vi "Keyboard MicroDrive Control.vi"() -> ()   [LabVIEW 2020]
uses:
  <vilib>/Utility/inputDevices.llb/keyboardAcquire.vi
  <vilib>/Utility/inputDevices.llb/closeKeyboard.vi
  MicroDrive.dll
panel:
  in  "Move size (um)":dbl=10.0
  in  "M3 Decreasing":string(combo)="16"
  in  "M3 Increasing":string(combo)="29"
  in  "Reset M3":bool
  out "M3-Encoder (um)":dbl format="%.3f"
  out "M3 Reverse Limit":bool
  out "M3 Forward Limit":bool
  in  "stop 2":bool
  in  "Stop":bool
  in  "Move":bool
  in  "Velocity (mm/s)":dbl=1.5 format="%.3f"
  in  "Keyboard Option":bool
  in  "M2 Increasing":string(combo)="32"
  in  "M2 Decreasing":string(combo)="28"
  in  "M1 Decreasing":string(combo)="10"
  in  "M1 Increasing":string(combo)="13"
  out "M1 Reverse Limit":bool
  out "M1 Forward Limit":bool
  out "M2 Reverse Limit":bool
  out "M2 Forward Limit":bool
  in  "Reset M2":bool
  out "M2-Encoder (um)":dbl format="%.3f"
  in  "Reset  All":bool
  in  "Reset M1":bool
  out "M1-Encoder (um)":dbl format="%.3f"
  in  "Move size (Um)":dbl=50.0 format="%.3f"
  in  "Axis":enum16{"M1", "M2", "M3"}(ring)
  in  "MoveMap":string(combo)="11"
  in  "HaltMap":string(combo)="12"
  out "First Key":T1(ring)
  out "keys pressed":T2(array[ring])
  out "Dir Ind":u32(knob) scale=0.0..36.0
  # "Encoder Monitor"
  # "Modified\nfor DM project"
  # "Options"
  # "Keyboard Configuration"
  # "Move without Keyboard"
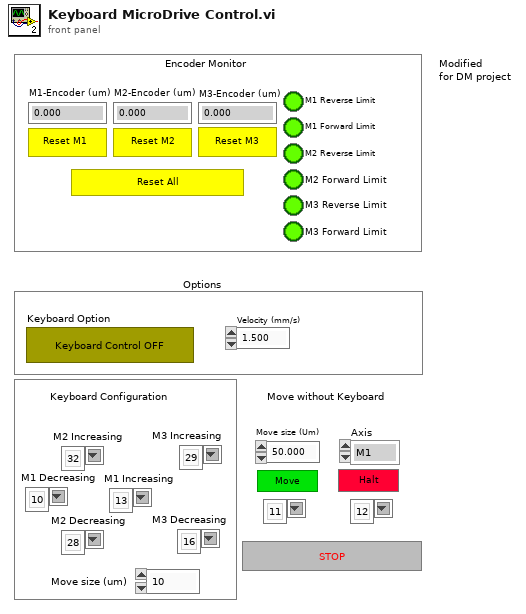
[diagram p1: front panel]
types:
  T1 = enum32{"0", "1", "2", "3", "4", "5", "6", "7", "8", "9", "A", "B", "C", "D", "E", "F", "G", "H", "I", "J", "K", "L", "M", "N", "O", "P", "Q", "R", "S", "T", "U", "V", "W", "X", "Y", "Z", "F1", "F2", "F3", "F4", "F5", "F6", "F7", "F8", "F9", "F10", "F11", "F12", "F13", "F14", "F15", "ADD", "BACK", "BACKSLASH", "CAPITAL", "COMMA", "DECIMAL", "DELETE", "DIVIDE", "DOWN", "END", "EQUALS", "ESCAPE", "GRAVE (`)", "HOME", "INSERT", "LBRACKET", "LCONTROL", "LEFT", "L ALT", "LSHIFT", "LWIN", "MINUS", "MULTIPLY", "NEXT", "NUMLOCK", "NUMPAD_0", "NUMPAD_1", "NUMPAD_2", "NUMPAD_3", "NUMPAD_4", "NUMPAD_5", "NUMPAD_6", "NUMPAD_7", "NUMPAD_8", "NUMPAD_9", "PAUSE", "PERIOD", "PRIOR (PG UP)", "RBRACKET", "RCONTROL", "RETURN", "RIGHT", "R ALT", "RSHIFT", "RWIN", "SCROLL", "SEMICOLON", "SLASH", "SPACE", "SUBTRACT", "TAB", "UP", "ENTER (num pad)", "' (quote)"}
  T2 = enum16{"0", "1", "2", "3", "4", "5", "6", "7", "8", "9", "A", "B", "C", "D", "E", "F", "G", "H", "I", "J", "K", "L", "M", "N", "O", "P", "Q", "R", "S", "T", "U", "V", "W", "X", "Y", "Z", "F1", "F2", "F3", "F4", "F5", "F6", "F7", "F8", "F9", "F10", "F11", "F12", "F13", "F14", "F15", "ADD", "BACK", "BACKSLASH", "CAPITAL", "COMMA", "DECIMAL", "DELETE", "DIVIDE", "DOWN", "END", "EQUALS", "ESCAPE", "GRAVE (`)", "HOME", "INSERT", "LBRACKET", "LCONTROL", "LEFT", "L ALT", "LSHIFT", "LWIN", "MINUS", "MULTIPLY", "NEXT", "NUMLOCK", "NUMPAD_0", "NUMPAD_1", "NUMPAD_2", "NUMPAD_3", "NUMPAD_4", "NUMPAD_5", "NUMPAD_6", "NUMPAD_7", "NUMPAD_8", "NUMPAD_9", "PAUSE", "PERIOD", "PRIOR (PG UP)", "RBRACKET", "RCONTROL", "RETURN", "RIGHT", "R ALT", "RSHIFT", "RWIN", "SCROLL", "SEMICOLON", "SLASH", "SPACE", "SUBTRACT", "TAB", "UP", "ENTER (num pad)", "' (quote)"}[]
  T3 = enum16{"0", "1", "2", "3", "4", "5", "6", "7", "8", "9", "A", "B", "C", "D", "E", "F", "G", "H", "I", "J", "K", "L", "M", "N", "O", "P", "Q", "R", "S", "T", "U", "V", "W", "X", "Y", "Z", "F1", "F2", "F3", "F4", "F5", "F6", "F7", "F8", "F9", "F10", "F11", "F12", "F13", "F14", "F15", "ADD", "BACK", "BACKSLASH", "CAPITAL", "COMMA", "DECIMAL", "DELETE", "DIVIDE", "DOWN", "END", "EQUALS", "ESCAPE", "GRAVE (`)", "HOME", "INSERT", "LBRACKET", "LCONTROL", "LEFT", "L ALT", "LSHIFT", "LWIN", "MINUS", "MULTIPLY", "NEXT", "NUMLOCK", "NUMPAD_0", "NUMPAD_1", "NUMPAD_2", "NUMPAD_3", "NUMPAD_4", "NUMPAD_5", "NUMPAD_6", "NUMPAD_7", "NUMPAD_8", "NUMPAD_9", "PAUSE", "PERIOD", "PRIOR (PG UP)", "RBRACKET", "RCONTROL", "RETURN", "RIGHT", "R ALT", "RSHIFT", "RWIN", "SCROLL", "SEMICOLON", "SLASH", "SPACE", "SUBTRACT", "TAB", "UP", "ENTER (num pad)", "' (quote)"}
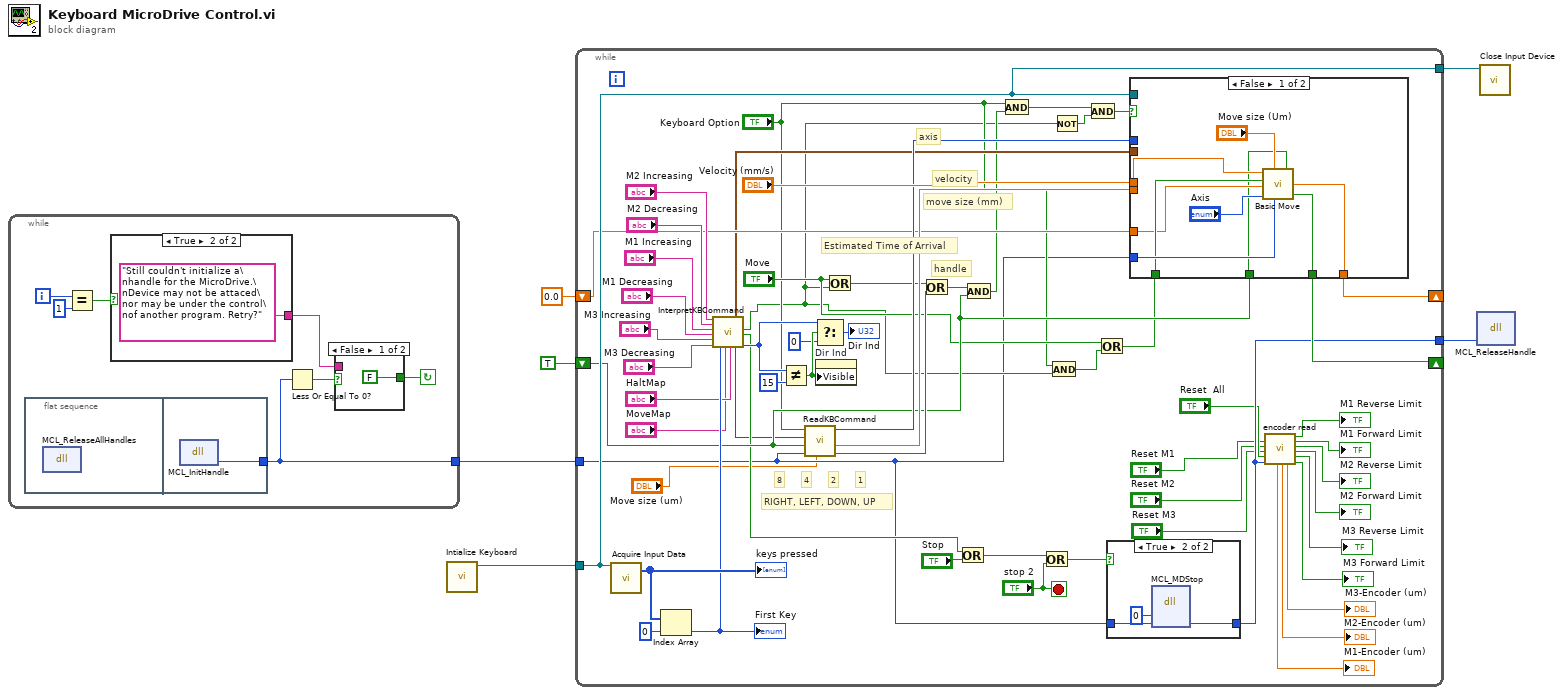
[diagram p0: block diagram]
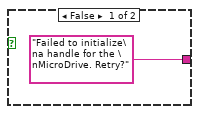
[diagram p2: hidden frame]
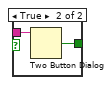
[diagram p3: hidden frame]
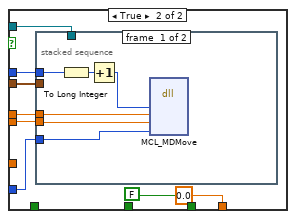
[diagram p4: hidden frame]
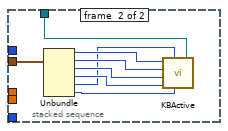
[diagram p5: hidden frame]
diagram:
  n1 = while {
    tunnel: [w13] -> w1
    i -> [w9]
    stop <- w10 continue-if-true
    n2 = flat-sequence {
      tunnel: [w19] -> w13
      frame #0 {
        n3 = dll-call lib="C:/Users/WalsworthGroup/Documents/Mad City Labs/MicroDrive/Labview Examples/MicroDrive.dll" fn="MCL_ReleaseAllHandles"() -> ()  [unwired: 3 in, 3 out]
      }
      frame #1 {
        n4 = dll-call lib="C:/Users/WalsworthGroup/Documents/Mad City Labs/MicroDrive/Labview Examples/MicroDrive.dll" fn="MCL_InitHandle" label="MicroDrive.dll:\nMCL_InitHandle"() -> ("handle"=w19:i32)  [unwired: 3 in, 2 out]
      }
    }
    n5 = Equal?(x=w9, y=1) -> (x = y?=w7:bool)
    n6 = case shown="True" w7 {
      tunnel: ["Failed to initialize\na handle for the \nMicroDrive. Retry?" ("message") "Still couldn't initialize a\nhandle for the MicroDrive.\nDevice may not be attaced\nor may be under the control\nof another program. Retry?" ("message")] -> w11
      frame False {
      }
      frame True {
      }
    }
    n7 = Less Or Equal To 0?(x=w13) -> (x <= 0?=w12:bool)
    n8 = case shown="False" w12 {
      tunnel: w11 -> [_ w18]
      tunnel: [FALSE ("T button?") w17] -> w10
      frame False {
      }
      frame True {
        n9 = Two Button Dialog(message=w18) -> (T button?=w17:bool)  [unwired: 2 out]
      }
    }
  }
  n10 = call <vilib>:"Intialize Keyboard.vi"() -> ("device ID"=w3:refnum<k1>)  [unwired: 1 in, 10 out]
  n11 = while {
    tunnel: w1 -> [w21]
    shift-right: [w59] -> _
    shift-left: TRUE -> [w57]
    shift-right: [w60] -> _
    shift-left: 0.0 -> [w58]
    tunnel: [w47] -> w4
    tunnel: w3 -> [w61]
    tunnel: [w61] -> w2
    stop <- "stop 2" stop-if-true
    # "8"
    # "4"
    # "2"
    # "1"
    # "RIGHT, LEFT, DOWN, UP"
    # "handle"
    # "axis"
    # "Estimated Time of Arrival"
    # "velocity"
    # "move size (mm)"
    n12 = call-poly <vilib>:"Acquire Input Data.vi"("device ID"=w61) -> ("keys pressed"=w74:T2)  [unwired: 1 in, 17 out]
    "keys pressed" <- w74
    n13 = Index Array "Index Array"(array=w74, index=0) -> (element=w62:T3)
    "First Key" <- w62
    n14 = call "InterpretKBCommand.vi"("M2 Increasing"="M2 Increasing", "M2 Decreasing"="M2 Decreasing", "M1 Increasing"="M1 Increasing", "M1 Decreasing"="M1 Decreasing", "M3 Increasing"="M3 Increasing", "M3 Decreasing"="M3 Decreasing", "Key\nValue"=w62, "MoveMap"="MoveMap", "HaltMap"="HaltMap") -> ("Cluster of Input #s"=w56:cluster{i32, i32, i32, i32, i32, i32}, "number"=w31:u32, "Move"=w22:bool, "Halt"=w48:bool, "Dir Indicator"=w54:u32)  [unwired: 6 out]
    n15 = Not Equal?(x=w54, y=u32 15 ("Dir Indicator")) -> (x != y?=w52:bool)
    n16 = call "ReadKBCommand.vi"("Move size (um)"="Move size (um)", "handle"=w21, "Feedback Disable\n(Enable = TRUE)"=w57, "Motion #"=w31, "Enable\n(True)"="Keyboard Option") -> ("Enable Move\n(TRUE)"=w69:bool, "Move size (mm)"=w70:dbl, "Axis"=w71:enum16{"X", "Y", "Z"})  [unwired: 4 in]
    n17 = Select(t=w54, s=w52, f=u32 0) -> (s? t:f=→"Dir Ind":u32)
    n18 = property on="Dir Ind" class="Knob (strict)"("Visible"=w52) -> ()  [unwired: 2 in, 2 out]
    n19 = Or(x="Move", y=w22) -> (x .or. y?=w50:bool)
    n20 = Or(x=w50, y=w69) -> (x .or. y?=w73:bool)
    n21 = Or(x=w48, y="Stop") -> (x .or. y?=w49:bool)
    n22 = And(x=w73, y=w57) -> (x .and. y?=w27:bool)
    n23 = And(x="Keyboard Option", y=w27) -> (x .and. y?=w30:bool)
    n24 = Or(x=w49, y="stop 2") -> (x .or. y?=w76:bool)
    n25 = And(x="Keyboard Option", y=w22) -> (x .and. y?=w24:bool)
    n26 = Not(x=w22) -> (.not. x?=w28:bool)
    n27 = And(x=w30, y=w28) -> (x .and. y?=w29:bool)
    n28 = Or(x="Move", y=w24) -> (x .or. y?=w26:bool)
    n29 = case shown="True" w76 {
      tunnel: w21 -> [w110 w112]
      tunnel: [w110 w111] -> w47
      frame False {
      }
      frame True {
        n30 = dll-call lib="C:/Users/WalsworthGroup/Documents/Mad City Labs/MicroDrive/Labview Examples/MicroDrive.dll" fn="MCL_MDStop" label="MicroDrive.dll:\nMCL_MDStop"("status"=u16 0, "handle"=w112) -> ("handle"=w111:i32)  [unwired: 3 in, 4 out]
      }
    }
    n31 = case shown="False" w29 {
      tunnel: w21 -> [w83 w88]
      tunnel: w71 -> [_ w95]
      tunnel: w70 -> [_ w93]
      tunnel: "Velocity (mm/s)" -> [w82 w94]
      tunnel: w61 -> [_ w92]
      tunnel: [w85 0.0 ("E.T.A.")] -> w60
      tunnel: [w84 FALSE ("Moving = False")] -> w59
      tunnel: w26 -> [w81 _]
      tunnel: w58 -> [w80 _]
      tunnel: w57 -> [w79 _]
      tunnel: w56 -> [_ w89]
      frame False {
        n32 = call "Basic Move.vi"("Velocity (mm/s)"=w82, "Move size (um)"="Move size (Um)", "Move = True"=w81, "Feedback E.T.A"=w80, "handle"=w83, "Axis"="Axis", "Feedback Moving"=w79) -> ("E.T.A."=w85:dbl, "Moving = False"=w84:bool)
      }
      frame True {
        n33 = stacked-sequence {
          tunnel: w95 -> [w99 _]
          tunnel: w94 -> [w98 _]
          tunnel: w88 -> [w97 _]
          tunnel: w93 -> [w96 _]
          tunnel: w92 -> [_ w109]
          tunnel: w89 -> [_ w108]
          frame #0 {
            n34 = To Long Integer(number=w99) -> (32bit integer=w101:i32)
            n35 = Increment(x=w101) -> (x+1=w100:i32)
            n36 = dll-call lib="C:/Users/WalsworthGroup/Documents/Mad City Labs/MicroDrive/Labview Examples/MicroDrive.dll" fn="MCL_MDMove" label="MicroDrive.dll:\nMCL_MDMove"("axis"=w100, "velocity"=w98, "distance"=w96, "handle"=w97) -> ()  [unwired: 7 in, 3 out]
          }
          frame #1 {
            n37 = Unbundle(w108) -> (w107:i32, w106:i32, w105:i32, w104:i32, w103:i32, w102:i32)
            n38 = call "KBActive.vi"("device ID"=w109, "M3 decreasing"=w102, "M3 increasing"=w103, "M1 increasing"=w104, "M1 decreasing"=w105, "M2 decreasing"=w106, "M2 increasing"=w107) -> ()
          }
        }
      }
    }
    n39 = call "encoder read.vi"("Reset M1"="Reset M1", "Reset M2"="Reset M2", "Reset M3"="Reset M3", "Reset  All"="Reset  All", "handle"=w47) -> ("M1-Encoder (um)"=→"M1-Encoder (um)":dbl, "M2-Encoder (um)"=→"M2-Encoder (um)":dbl, "M3-Encoder (um)"=→"M3-Encoder (um)":dbl, "M1 Reverse Limit"=→"M1 Reverse Limit":bool, "M1 Forward Limit"=→"M1 Forward Limit":bool, "M2 Reverse Limit"=→"M2 Reverse Limit":bool, "M2 Forward Limit"=→"M2 Forward Limit":bool, "M3 Reverse Limit"=→"M3 Reverse Limit":bool, "M3 Forward Limit"=→"M3 Forward Limit":bool)  [unwired: 6 in]
  }
  n40 = dll-call lib="C:/Users/WalsworthGroup/Documents/Mad City Labs/MicroDrive/Labview Examples/MicroDrive.dll" fn="MCL_ReleaseHandle" label="MicroDrive.dll:\nMCL_ReleaseHandle"("handle"=w4) -> ()  [unwired: 4 in, 3 out]
  n41 = call-poly <vilib>:"Close Input Device.vi"("device ID"=w2) -> ()  [unwired: 1 in, 9 out]
